vi "report_config.vi"(8 "error in (no error)":errorcluster, 10 "Cluster":T1, 11 "Instrument in":refnum<class "Instrument.lvclass">) -> (0 "error out":errorcluster, 3 "Instrument out":refnum<class "Instrument.lvclass">)   [LabVIEW 2019, in "Instrument.lvclass"]
uses:
  Instrument.lvclass
  core/core_reportCfg.ctl
  core/core_reportMode.ctl
  Instrument.lvclass/Instrument.ctl
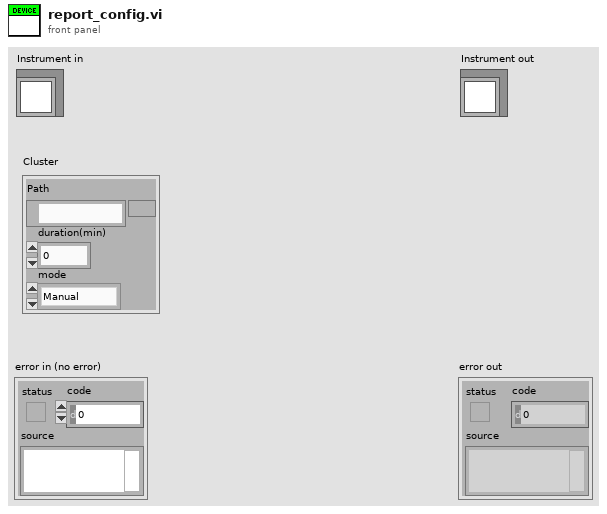
[diagram p1: front panel]
types:
  T1 = typedef "core_reportCfg.ctl" = cluster{"Path":path, "duration(min)":i32, "mode":T2}
  T2 = typedef "core_reportMode.ctl" = enum16{"Manual", "Automatic"}
  T3 = enum16{"open", "replace", "create", "open or create", "replace or create", "replace or create with confirmation"}
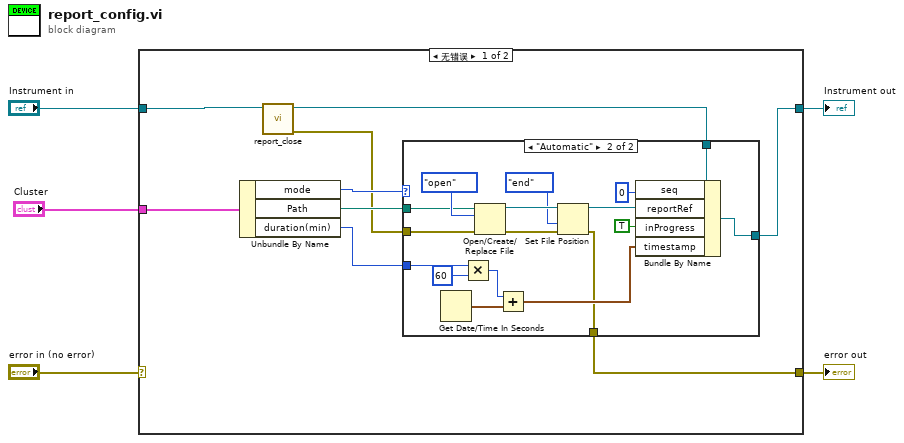
[diagram p0: block diagram]
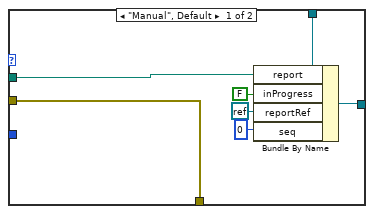
[diagram p2: hidden frame]
diagram:
  n1 = case shown="无错误" "error in (no error)" {
    selector: "error in (no error)" -> [_ w40]
    tunnel: [w9 w40] -> w4
    tunnel: [w10 w39] -> w2
    tunnel: "Instrument in" -> [w8 w39]
    tunnel: "Cluster" -> [w14 _]
    frame No Error {
      n2 = Unbundle By Name(w14) -> ("mode"=w13:T2, "Path"=w12:path, "duration(min)"=w11:i32)
      n3 = call "report_close.vi"("Instrument in"=w8) -> ("error out"=w6:errorcluster, "Instrument out"=w7:refnum<class "Instrument.lvclass">)  [unwired: 9 in]
      n4 = case shown="\"Automatic\"" w13 {
        tunnel: w7 -> [w21 w38]
        tunnel: w12 -> [w16 w28]
        tunnel: w11 -> [_ w33]
        tunnel: [w15 w24] -> w9
        tunnel: [w18 w29] -> w10
        tunnel: w6 -> [w15 w22]
        frame "Manual", Default {
          n5 = Bundle By Name(cluster=w21, "report"=w16, "inProgress"=FALSE, "reportRef"=refnum<k0> refnum, "seq"=0) -> (w18:refnum<class "Instrument.lvclass">)
        }
        frame "Automatic" {
          n6 = Get Date/Time In Seconds() -> (seconds since 1Jan1904=w34:timestamp)
          n7 = Multiply(x=w33, y=60) -> (x*y=w31:i32)
          n8 = Open/Create/Replace File(file path (use dialog)=w28, error in=w22, operation (0:open)=T3."open") -> (refnum out=w37:refnum<file>, error out=w25:errorcluster)  [unwired: 3 in, 1 out]
          n9 = Add(x=w31, y=w34) -> (x+y=w30:timestamp)
          n10 = Set File Position(refnum=w37, from (0:start)=enum16{"start", "end", "current"}."end", error in=w25) -> (refnum out=w26:refnum<file>, error out=w24:errorcluster)  [unwired: 1 in]
          n11 = Bundle By Name(cluster=w38, "seq"=0, "reportRef"=w26, "inProgress"=TRUE, "timestamp"=w30) -> (w29:refnum<class "Instrument.lvclass">)
        }
      }
    }
    frame Error {
    }
  }
  "error out" <- w4
  "Instrument out" <- w2
